vi "Add content to Engine library.vi"(6 "Project Name":string, 8 "error in (no error)":errorcluster, 9 "Project Root":path, 10 "CD Wizard - Internal Data":T1, 11 "CD Template":refnum<class "NIVS_PPL_Inline HW Interface.lvclass">) -> (0 "error out":errorcluster)   [LabVIEW 2019, in "NIVS_PPL_Inline HW Interface.lvclass"]
doc: "Add all virtual folders and VIs to the Engine library."
uses:
  NIVS_PPL_Inline HW Interface.lvclass
  NIVS_Consolidated_CDW_MetaDataObj/Internal data.ctl
  NIVS_Consolidated_CDW_MetaDataObj/CD Engine lvlib.ctl
  NIVS_Consolidated_CDW_MetaDataObj/Add Item - Type.ctl
  NIVS_Consolidated_CDW_MetaDataObj/CD Engine lvlib.vi
  NIVS_Consolidated_CDW_MetaDataObj/NIVS_Consolidated_CDW_MetaDataObj.lvclass
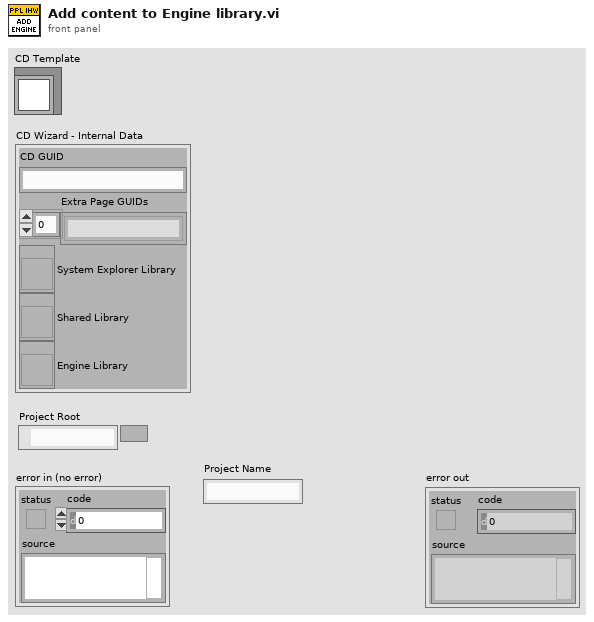
[diagram p1: front panel]
types:
  T1 = typedef "NIVS_Consolidated_CDW_MetaDataObj.lvclass/Internal data.ctl" = cluster{"CD GUID":string, "Extra Page GUIDs":string[], "System Explorer Library":refnum<vi>, "Shared Library":refnum<vi>, "Engine Library":refnum<vi>}
  T2 = typedef "NIVS_Consolidated_CDW_MetaDataObj.lvclass/CD Engine lvlib.ctl" = enum16{"LibraryFileName", "LibraryFolderName", "Engine.FolderName", "Engine.Init.FolderName", "Engine.Run.FolderName", "Engine.Shutdown.FolderName", "Types.FolderName", "Engine.RT Driver VI.TemplatePath", "Engine.RT Driver VI.FileName", "Engine.PPL.RT Driver VI_InlineAsync.FileName", "Engine.RTStateVariables.Name", "Engine.PPL.RTStateVariables.Name", "Engine.RTStateVariables.Name.NoExtension", "Engine.Async.NameExtension", "Engine.Async.TemplateName", "Engine.PPL.Async.TemplateName", "Engine.PPL.Async.InitVSGlobals.Name", "Engine.PPL.RT Driver VI_Inline.FileName"}
  T3 = typedef "NIVS_Consolidated_CDW_MetaDataObj.lvclass/Add Item - Type.ctl" = string
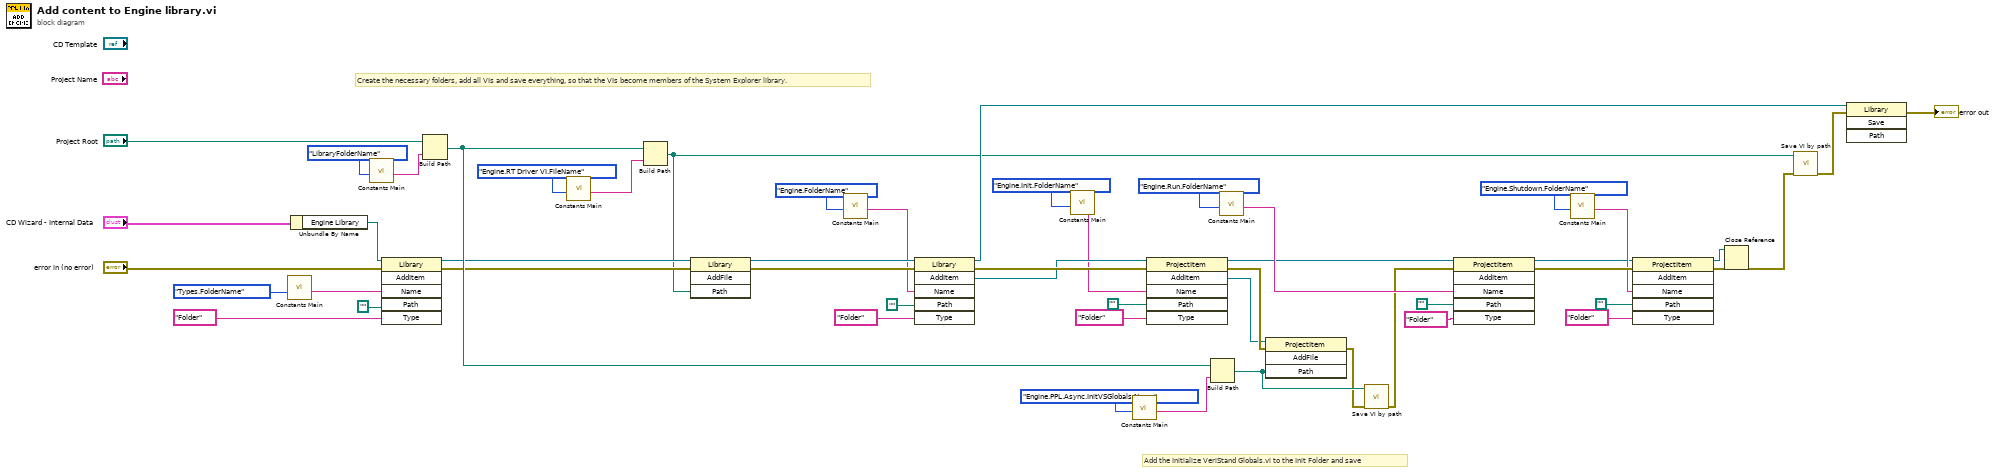
[diagram p0: block diagram]
diagram:
  # "Add the Initialize VeriStand Globals.vi to the Init Folder and save"
  # "Create the necessary folders, add all VIs and save everything, so that the VIs become members of the System Explorer library."
  n1 = call-poly "Constants Main.vi"("Action"=CD_Engine_lvlib."Types.FolderName") -> ("Output"=w10:string)  [unwired: 10 in]
  n2 = Unbundle By Name("CD Wizard - Internal Data") -> ("Engine Library"=w19:refnum<vi>)
  n3 = call-poly "Constants Main.vi"("Action"=CD_Engine_lvlib."LibraryFolderName") -> ("Output"=w17:string)  [unwired: 10 in]
  n4 = invoke class="Library" method="AddItem"(reference=w19, error in="error in (no error)", "Name"=w10, "Path"=path "", "Type"=T3 "Folder" ("Add Item - Type")) -> (reference out=w44:refnum<vi>, error out=w43:errorcluster)  [unwired: 1 in, 4 out]
  n5 = Build Path(base path="Project Root", name or relative path=w17) -> (appended path=w48:path)
  n6 = call-poly "Constants Main.vi"("Action"=CD_Engine_lvlib."Engine.RT Driver VI.FileName") -> ("Output"=w15:string)  [unwired: 10 in]
  n7 = Build Path(base path=w48, name or relative path=w15) -> (appended path=w36:path)
  n8 = invoke class="Library" method="AddFile"(reference=w44, error in=w43, "Path"=w36) -> (reference out=w24:refnum<vi>, error out=w45:errorcluster)  [unwired: 1 in, 2 out]
  n9 = call-poly "Constants Main.vi"("Action"=CD_Engine_lvlib."Engine.FolderName") -> ("Output"=w22:string)  [unwired: 10 in]
  n10 = invoke class="Library" method="AddItem"(reference=w24, error in=w45, "Name"=w22, "Path"=path "", "Type"=T3 "Folder" ("Add Item - Type")) -> (reference out=w37:refnum<vi>, error out=w46:errorcluster, "AddItem"=w25:refnum<vi>)  [unwired: 1 in, 3 out]
  n11 = call-poly "Constants Main.vi"("Action"=CD_Engine_lvlib."Engine.Init.FolderName") -> ("Output"=w14:string)  [unwired: 10 in]
  n12 = call-poly "Constants Main.vi"("Action"=CD_Engine_lvlib."Engine.PPL.Async.InitVSGlobals.Name") -> ("Output"=w49:string)  [unwired: 10 in]
  n13 = invoke class="ProjectItem" method="AddItem"(reference=w25, error in=w46, "Name"=w14, "Path"=path "", "Type"=T3 "Folder" ("Add Item - Type")) -> (reference out=w27:refnum<vi>, error out=w51:errorcluster, "AddItem"=w50:refnum<vi>)  [unwired: 1 in, 3 out]
  n14 = Build Path(base path=w48, name or relative path=w49) -> (appended path=w52:path)
  n15 = call-poly "Constants Main.vi"("Action"=CD_Engine_lvlib."Engine.Run.FolderName") -> ("Output"=w29:string)  [unwired: 10 in]
  n16 = invoke class="ProjectItem" method="AddFile"(reference=w50, error in=w51, "Path"=w52) -> (error out=w2:errorcluster)  [unwired: 1 in, 3 out]
  n17 = call "Save VI by path.vi"("error in (no error)"=w2, "VI path"=w52) -> ("error out"=w1:errorcluster)  [unwired: 9 in]
  n18 = invoke class="ProjectItem" method="AddItem"(reference=w27, error in=w1, "Name"=w29, "Path"=path "", "Type"=T3 "Folder" ("Add Item - Type")) -> (reference out=w35:refnum<vi>, error out=w42:errorcluster)  [unwired: 1 in, 4 out]
  n19 = call-poly "Constants Main.vi"("Action"=CD_Engine_lvlib."Engine.Shutdown.FolderName") -> ("Output"=w38:string)  [unwired: 10 in]
  n20 = invoke class="ProjectItem" method="AddItem"(reference=w35, error in=w42, "Name"=w38, "Path"=path "", "Type"=T3 "Folder" ("Add Item - Type")) -> (reference out=w41:refnum<vi>, error out=w39:errorcluster)  [unwired: 1 in, 4 out]
  n21 = Close Reference(reference=w41, error in (no error)=w39) -> (error out=w40:errorcluster)
  n22 = call "Save VI by path.vi"("error in (no error)"=w40, "VI path"=w36) -> ("error out"=w8:errorcluster)  [unwired: 9 in]
  n23 = invoke class="Library" method="Save"(reference=w37, error in=w8) -> (error out=→"error out":errorcluster)  [unwired: 2 in, 3 out]
